vi "UART Read.vi"   [LabVIEW 2020, in "LMH-LINX.lvlib"]
uses:
  LMH-LINX.lvlib
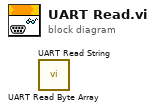
[diagram p0: block diagram]
diagram:
  n1 = call "UART Read Byte Array.vi"() -> ()  [unwired: 9 in, 3 out]
  n2 = call "UART Read String.vi"() -> ()  [unwired: 9 in, 3 out]
